vi "Software Update HCC Rename Latest EXE.vi"(8 "error in (no error)":errorcluster, 10 "Latest Exe Files":path[](array[path]), 11 "Path Build List Sub Input":path) -> (0 "error out":errorcluster, 2 "Array":path[](array[path]))   [LabVIEW 2016]
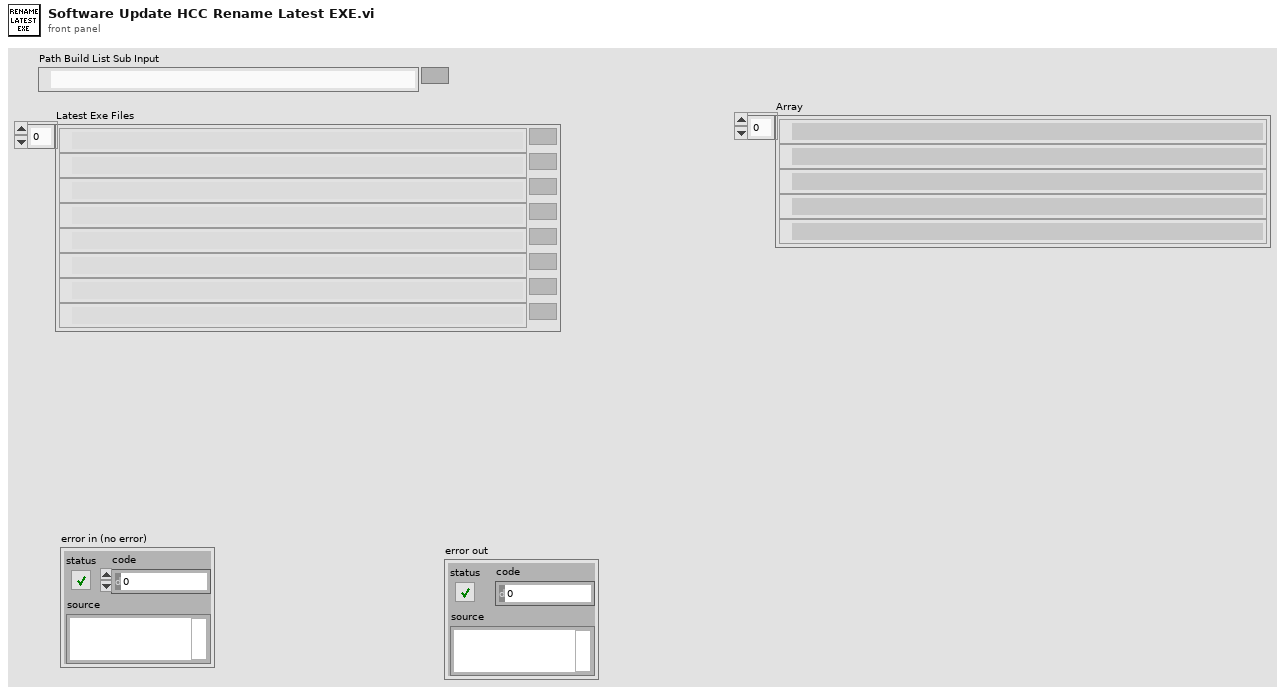
[diagram p1: front panel]
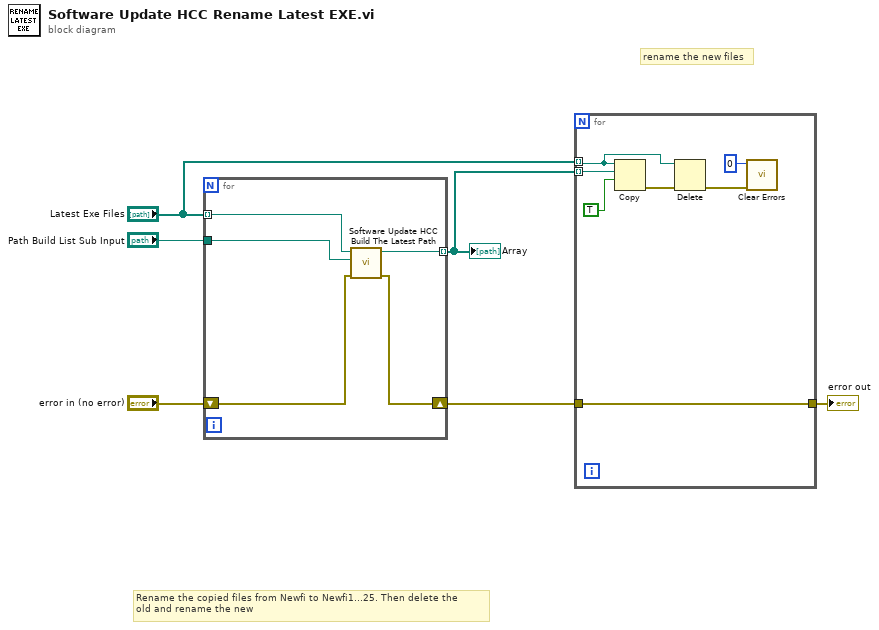
[diagram p0: block diagram]
diagram:
  # "rename the new files"
  # "Rename the copied files from Newfi to Newfi1...25. Then delete the\nold and rename the new"
  n1 = for {
    tunnel: "Latest Exe Files" -> [w10] mode=indexing
    tunnel: "Path Build List Sub Input" -> [w11]
    shift-right: [w7] -> w2
    shift-left: "error in (no error)" -> [w8]
    tunnel: [w9] -> w4 mode=indexing
    n2 = call "Software Update HCC Build The Latest Path.vi"("Error In"=w8, "Path Build List Sub Input"=w11, "Latest Exe Files"=w10) -> ("Error Out"=w7:errorcluster, "Updated Path"=w9:path)  [unwired: 7 in]
  }
  "Array" <- w4
  n3 = for {
    tunnel: w4 -> [w15] mode=indexing
    tunnel: "Latest Exe Files" -> [w12] mode=indexing
    tunnel: w2 -> [w13]
    tunnel: [w13] -> w1
    n4 = Copy(9:TRUE ("overwrite (F)"), 10:w15, 11:w12) -> (0:w16:errorcluster)  [unwired: 2 in, 2 out]
    n5 = Delete(path (use dialog)=w12, error in=w16) -> (error out=w17:errorcluster)  [unwired: 3 in, 2 out]
    n6 = call <vilib>:"Clear Errors.vi"("error in (no error)"=w17, "specific error code to clear (0: all)"=0) -> ()  [unwired: 4 in, 2 out]
  }
  "error out" <- w1
